vi "myRIO_BRig_Host_test_dataGeneration_inputConditions.vi"(10 "nTrial_perBlock":u16, 11 "input_nTrial_total":u16) -> (2 "output_nTrial_perBlock":u16, 3 "output_nTrial_total":u16)   [LabVIEW 2014]
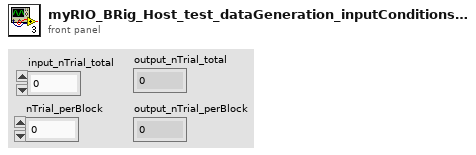
[diagram p1: front panel]
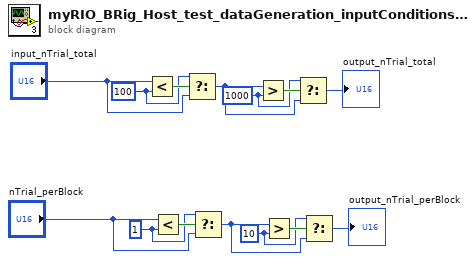
[diagram p0: block diagram]
diagram:
  w3 = u16 10 ("y")
  w6 = u16 1 ("y")
  w9 = u16 1000 ("y")
  w12 = u16 100 ("y")
  n1 = Less?(x="input_nTrial_total", y=w12) -> (x < y?=w14:bool)
  n2 = Less?(x="nTrial_perBlock", y=w6) -> (x < y?=w7:bool)
  n3 = Select(t=w12, s=w14, f="input_nTrial_total") -> (s? t:f=w10:u16)
  n4 = Select(t=w6, s=w7, f="nTrial_perBlock") -> (s? t:f=w4:u16)
  n5 = Greater?(x=w10, y=w9) -> (0:w11:bool)
  n6 = Greater?(x=w4, y=w3) -> (0:w5:bool)
  n7 = Select(t=w9, s=w11, f=w10) -> (s? t:f=→"output_nTrial_total":u16)
  n8 = Select(t=w3, s=w5, f=w4) -> (s? t:f=→"output_nTrial_perBlock":u16)
